vi "Unsubscribe SensorView.vi"(8 "error in (no error)":errorcluster, 10 "SensorView Enqueuer":refnum<class "Message Enqueuer.lvclass">, 11 "Sensor in":refnum<class "Sensor.lvclass">) -> (0 "error out":errorcluster, 3 "Sensor out":refnum<class "Sensor.lvclass">)   [LabVIEW 2012, in "Sensor Definition.lvlib" / "Sensor.lvclass"]
uses:
  Sensor.lvclass
  <vilib>/ActorFramework/Message Enqueuer/Message Enqueuer.lvclass
  <vilib>/ActorFramework/Actor/Actor.lvclass/Actor.ctl
  Sensor.lvclass/Sensor.ctl
  <vilib>/ActorFramework/Message Enqueuer/Message Enqueuer.lvclass/Message Enqueuer.ctl
  Read Listening SensorViews.vi
  Read Listening HostTypes.vi
  Write Listening SensorViews.vi
  Write Listening HostTypes.vi
  <vilib>/ActorFramework/Message Enqueuer/Enqueue.vi
  <vilib>/ActorFramework/Message Priority Queue/Priority Enqueue.vi
  Win8uiFramework/MainController Messages/MainPane SubView Exit Msg/MainPane SubView Exit Msg.lvclass
  <vilib>/ActorFramework/Actor/Actor.lvclass
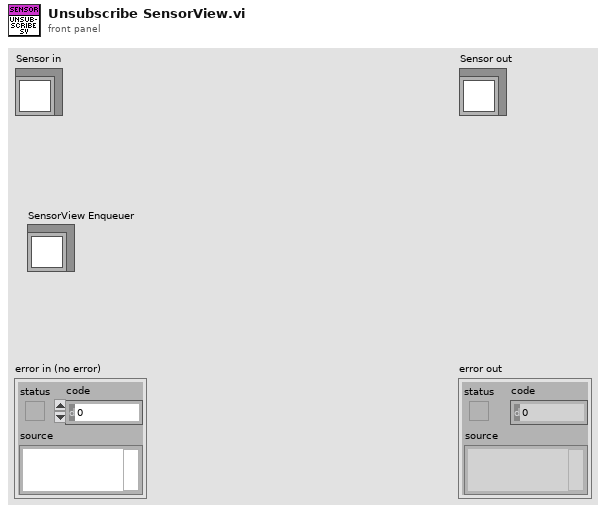
[diagram p1: front panel]
types:
  T1 = typedef "Sensor Definition.lvlib/HostType.ctl" = enum16{"Standalone", "Grid", "MainPane"}
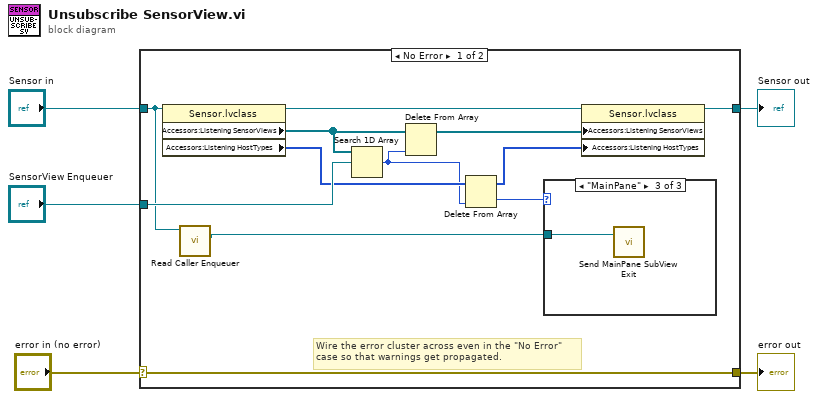
[diagram p0: block diagram]
diagram:
  n1 = case shown="No Error" "error in (no error)" {
    selector: "error in (no error)" -> [w17 w20]
    tunnel: [w17 w20] -> w4
    tunnel: [w15 w19] -> w2
    tunnel: "Sensor in" -> [w7 w19]
    tunnel: "SensorView Enqueuer" -> [w14 _]
    frame No Error {
      # "Wire the error cluster across even in the \"No Error\"\ncase so that warnings get propagated."
      n2 = property class="Sensor.lvclass"(reference=w7) -> (reference out=w16:refnum<class "Sensor.lvclass">, "Accessors:Listening SensorViews"=w13:refnum<class "Message Enqueuer.lvclass">[], "Accessors:Listening HostTypes"=w11:T1[])  [unwired: 1 in, 1 out]
      n3 = call <vilib>:"Read Caller Enqueuer.vi"("Actor"=w7) -> ("Caller Enqueuer"=w6:refnum<class "Message Enqueuer.lvclass">)  [unwired: 10 in]
      n4 = Search 1D Array(1D array=w13, element=w14) -> (index of element=w9:i32)  [unwired: 1 in]
      n5 = Delete From Array(array=w13, index=w9) -> (array with subset deleted=w12:refnum<class "Message Enqueuer.lvclass">[])  [unwired: 1 in, 1 out]
      n6 = Delete From Array(array=w11, index=w9) -> (deleted portion=w8:T1, array with subset deleted=w10:T1[])  [unwired: 1 in]
      n7 = case shown="\"MainPane\"" w8 {
        tunnel: w6 -> [_ _ w18]
        frame "Standalone", Default {
        }
        frame "Grid" {
        }
        frame "MainPane" {
          n8 = call "Send MainPane SubView Exit.vi"("Message Enqueuer"=w18) -> ()  [unwired: 9 in, 2 out]
        }
      }
      n9 = property class="Sensor.lvclass"(reference=w16, "Accessors:Listening SensorViews"=w12, "Accessors:Listening HostTypes"=w10) -> (reference out=w15:refnum<class "Sensor.lvclass">)  [unwired: 1 in, 1 out]
    }
    frame Error {
    }
  }
  "error out" <- w4
  "Sensor out" <- w2
